vi "Dist to Ticks.vi"(8 "error in (no error)":errorcluster, 10 "distance (m)":dbl, 11 "KUKA youBot gripper motor_EtherCAT in":refnum<class "NI_Robotics_KUKA youBot Gripper Motor_EtherCAT.lvclass">) -> (0 "error out":errorcluster, 2 "ticks":i32, 3 "KUKA youBot gripper motor_EtherCAT out":refnum<class "NI_Robotics_KUKA youBot Gripper Motor_EtherCAT.lvclass">)   [LabVIEW 2017, in "NI_Robotics_KUKA youBot Host.lvlib" / "NI_Robotics_KUKA youBot Gripper Motor_EtherCAT.lvclass"]
uses:
  <vilib>/robotics/KUKA youBot/Motor/Gripper Motor EtherCAT/NI_Robotics_KUKA youBot Gripper Motor_EtherCAT.lvclass
  <vilib>/robotics/KUKA youBot/Motor/Gripper Motor EtherCAT/NI_Robotics_KUKA youBot Gripper Motor_EtherCAT.lvclass/NI_Robotics_KUKA youBot Gripper Motor_EtherCAT.ctl
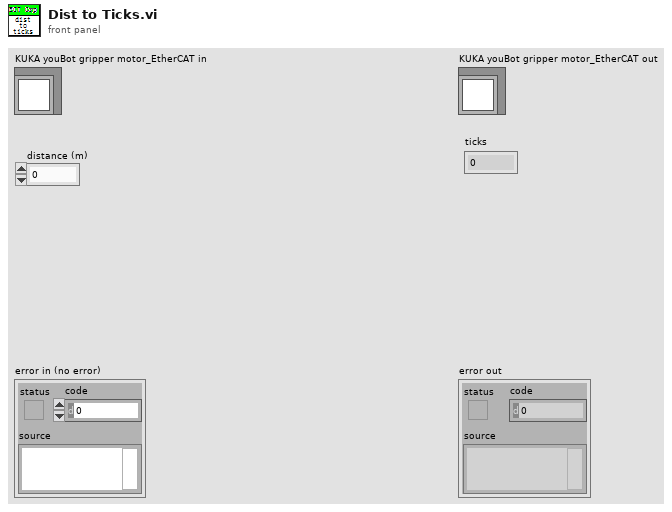
[diagram p1: front panel]
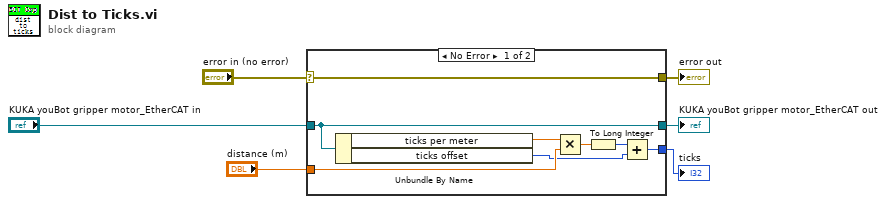
[diagram p0: block diagram]
diagram:
  n1 = case shown="No Error" "error in (no error)" {
    selector: "error in (no error)" -> [w14 w16]
    tunnel: [w14 w16] -> w5
    tunnel: [w13 w15] -> w3
    tunnel: "KUKA youBot gripper motor_EtherCAT in" -> [w13 w15]
    tunnel: "distance (m)" -> [w11 _]
    tunnel: [w9 _] -> w1
    frame No Error {
      n2 = Unbundle By Name(w13) -> ("ticks per meter"=w12:dbl, "ticks offset"=w10:i32)
      n3 = Multiply(x=w12, y=w11) -> (x*y=w8:dbl)
      n4 = To Long Integer(number=w8) -> (32bit integer=w7:i32)
      n5 = Add(x=w7, y=w10) -> (x+y=w9:i32)
    }
    frame Error {
    }
  }
  "error out" <- w5
  "KUKA youBot gripper motor_EtherCAT out" <- w3
  "ticks" <- w1
